vi "string to bytes (SubVI).vi"(10 "String":string) -> (2 "unsigned byte array":u8[](array[numeric]))   [LabVIEW 2021]
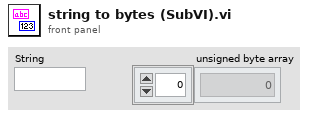
[diagram p1: front panel]
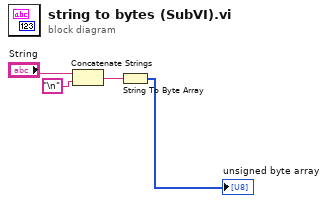
[diagram p0: block diagram]
diagram:
  n1 = Concatenate Strings("String", "\n") -> (w3:string)
  n2 = String To Byte Array(string=w3) -> (unsigned byte array=→"unsigned byte array":u8[])
